vi "gsp_simulator_release.vi"(4 "error in (no error)":errorcluster) -> (0 "error out":errorcluster)   [LabVIEW 2015]
doc: "Release the serial port"
uses:
  gsp_simulator_global.vi
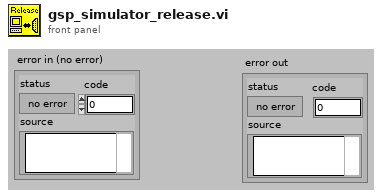
[diagram p1: front panel]
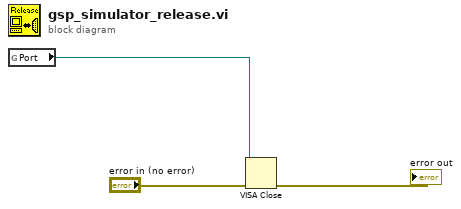
[diagram p0: block diagram]
diagram:
  n1 = global read "gsp_simulator_global.vi" "Port"() -> (w3:refnum<visa-resource-name>)
  n2 = VISA Close(VISA resource name=w3, error in (no error)="error in (no error)") -> (error out=→"error out":errorcluster)
